vi "XVC_TX.vi"(6 "data in":string, 7 "Read (TRUE)":bool, 8 "error in":errorcluster, 9 "Address":u32=2056 format="%.0x", 10 "IP address":string="192.168.10.20", 11 "connection ID":refnum<k16>) -> (0 "error out":errorcluster, 2 "received string":string, 3 "connection ID 2":refnum<k16>)   [LabVIEW 2017]
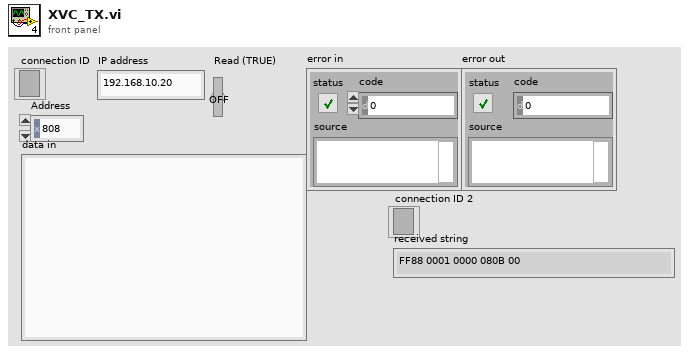
[diagram p1: front panel]
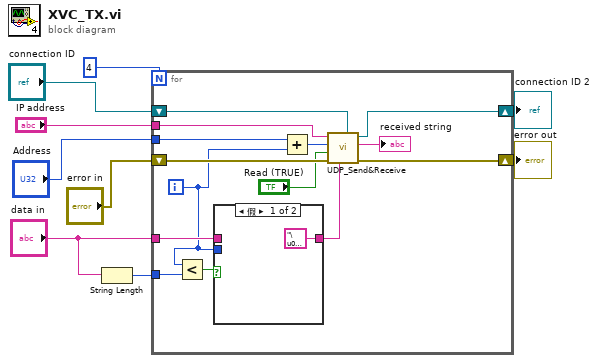
[diagram p0: block diagram]
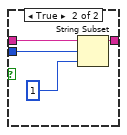
[diagram p2: hidden frame]
diagram:
  n1 = String Length(string="data in") -> (length=w1:i32)
  n2 = for {
    N: 4 -> [_]
    shift-right: [w22] -> w4
    shift-left: "connection ID" -> [w23]
    tunnel: "Address" -> [w20]
    tunnel: "data in" -> [w19]
    shift-right: [w17] -> w5
    shift-left: "error in" -> [w16]
    tunnel: "IP address" -> [w15]
    tunnel: w1 -> [w11]
    i -> [w10]
    n3 = Less?(x=w10, y=w11) -> (x < y?=w12:bool)
    n4 = case shown="假" w12 {
      tunnel: w19 -> [_ w28]
      tunnel: ["\u0000" ("data in") w27] -> w18
      tunnel: w10 -> [_ w25]
      frame False {
      }
      frame True {
        n5 = String Subset(string=w28, offset (0)=w25, length (rest)=1 ("length (rest)")) -> (substring=w27:string)
      }
    }
    n6 = Add(x=w20, y=w10) -> (x+y=w21:u32)
    n7 = call "UDP_Send&Receive.vi"("connection ID"=w23, "In"=w18, "error in (no error)"=w16, "Read (TRUE)"="Read (TRUE)", "Address"=w21, "IP address"=w15) -> ("error out"=w17:errorcluster, "received string"=→"received string":string, "connection ID out"=w22:refnum<k16>)  [unwired: 1 in, 1 out]
  }
  "error out" <- w5
  "connection ID 2" <- w4
